vi "Write Micron Optics Driver.vi"(8 "error in (no error)":errorcluster, 10 "Micron Optics Driver.lvclass":refnum<class "Micron Optics Driver.lvclass">, 11 "Micron Optics Recorder in":refnum<class "Micron Optics Recorder.lvclass">) -> (0 "error out":errorcluster, 3 "Micron Optics Recorder out":refnum<class "Micron Optics Recorder.lvclass">)   [LabVIEW 2016, in "Micron Optics Recorder.lvclass"]
uses:
  Micron Optics Recorder.lvclass
  C:/github/LabActor/Instrument Actor/Instrument Actor.lvclass
  NHMFL_Core/Libraries/Instruments/Micron Optics/Micron Optics Driver/Micron Optics Driver.lvclass
  C:/github/NHMFL_Core/Libraries/Instruments/Instrument Driver/Instrument Driver.lvclass
  Instrument Actor/Instrument Actor.lvclass/Instrument Actor.ctl
  Instrument Actor/Write Instrument driver.vi
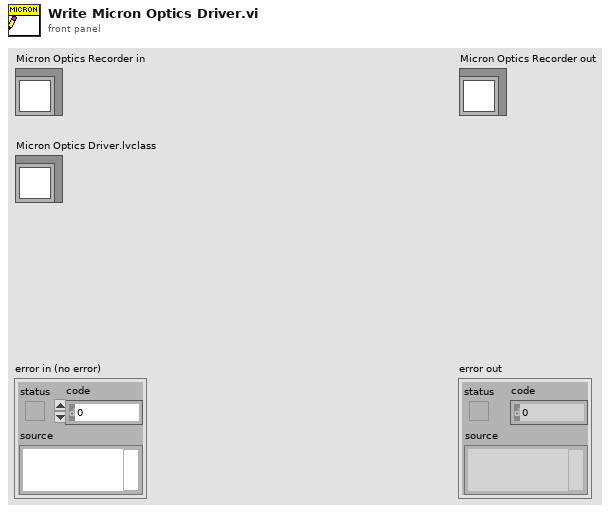
[diagram p1: front panel]
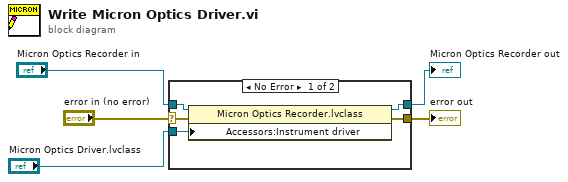
[diagram p0: block diagram]
diagram:
  n1 = case shown="No Error" "error in (no error)" {
    selector: "error in (no error)" -> [w10 w11]
    tunnel: [w9 w11] -> w4
    tunnel: [w7 w12] -> w2
    tunnel: "Micron Optics Recorder in" -> [w8 w12]
    tunnel: "Micron Optics Driver.lvclass" -> [w6 _]
    frame No Error {
      n2 = property class="Micron Optics Recorder.lvclass"(reference=w8, error in=w10, "Accessors:Instrument driver"=w6) -> (reference out=w7:refnum<class "Micron Optics Recorder.lvclass">, error out=w9:errorcluster)
    }
    frame Error {
    }
  }
  "error out" <- w4
  "Micron Optics Recorder out" <- w2
